vi "Waaagh_ProcessImage_Binary.vi"() -> ()   [LabVIEW 2016]
uses:
  <vilib>/vision/NI_Vision_Development_Module.lvlib
panel:
  out "Image 2":T1(plugin-control)
  out "Image":T1(plugin-control)
  in  "stop":bool
  in  "Binary":string
  in  "Range":cluster{"Lower value":sgl, "Upper value":sgl}={"Lower value"=128.0, "Upper value"=255.0} {"Upper value" format="%.2f"; "Lower value" format="%.2f"}
  in  "File Path":path
  in  "String":string
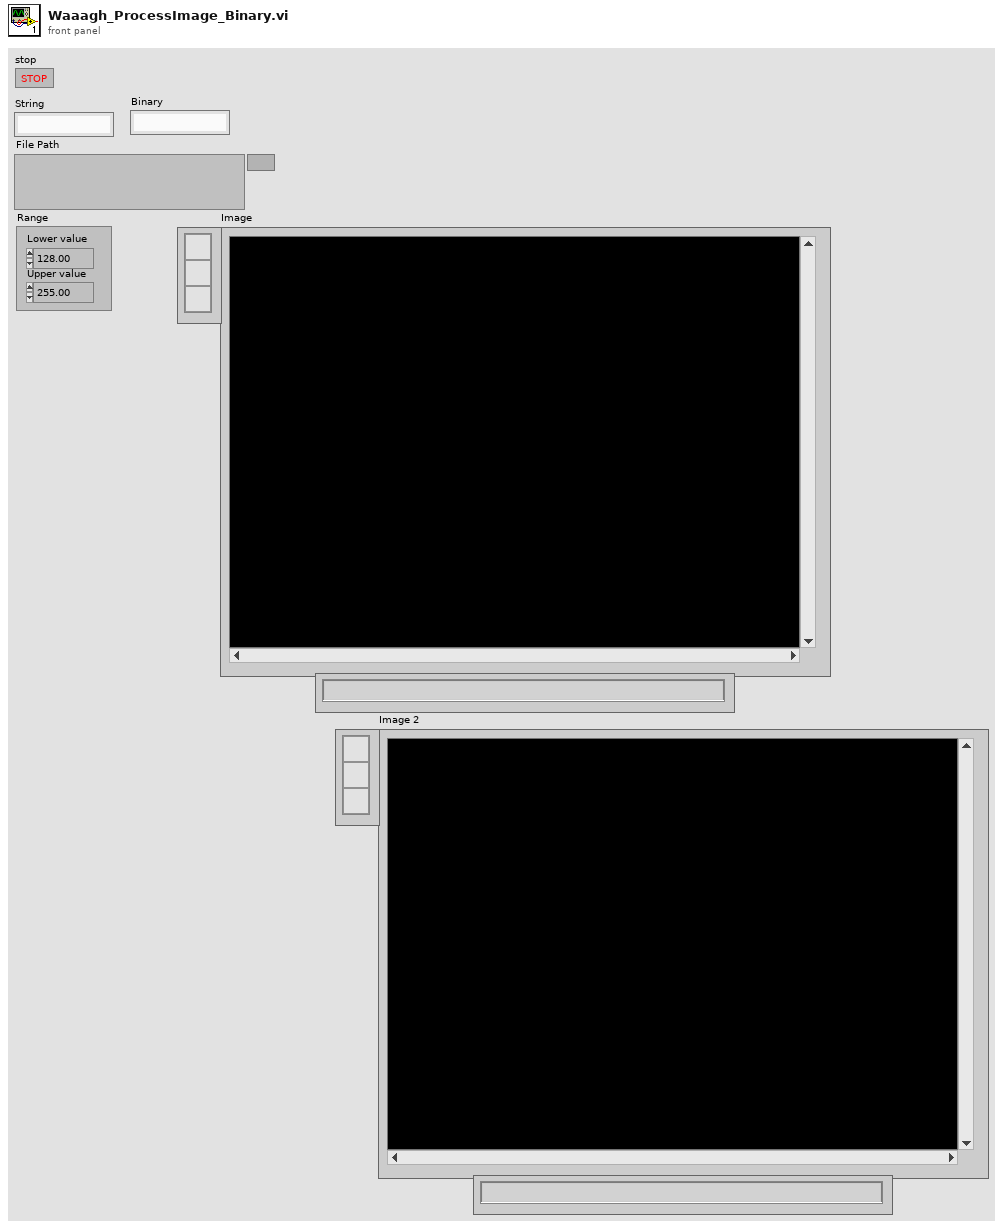
[diagram p1: front panel]
types:
  T1 = typedef "IMAQ Image.ctl" = refnum<image>
  T2 = typedef "Image Type" = u32
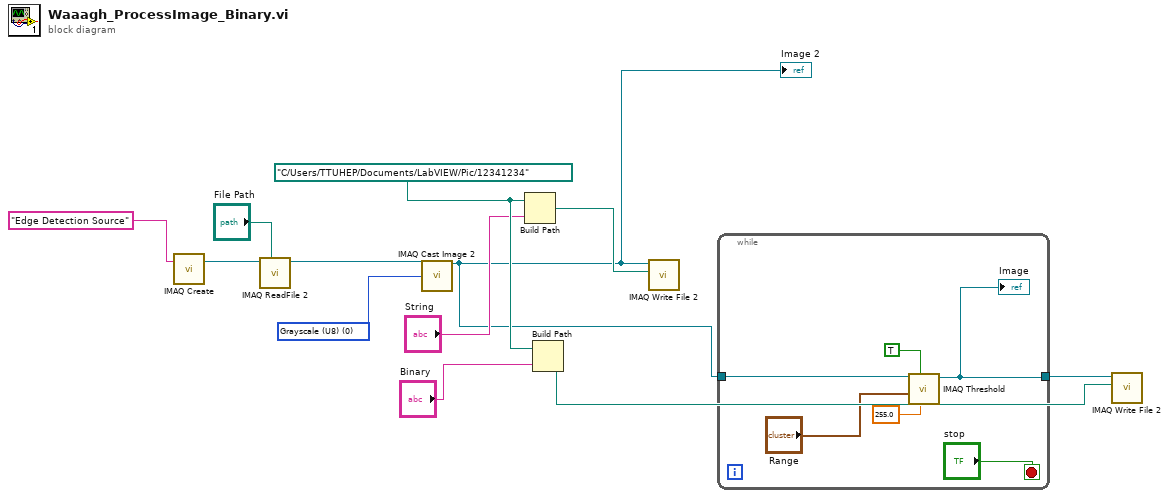
[diagram p0: block diagram]
diagram:
  w6 = path "C:/Users/TTUHEP/Documents/LabVIEW/Pic/12341234"
  w12 = T2 0 items=["Grayscale (U8)", "Grayscale (I16)", "Grayscale (SGL)", "Complex (CSG)", "RGB (U32)", "HSL (U32)", "RGB (U64)", "Grayscale (U16)"] ("Image Type")
  n1 = call "IMAQ Create"("Image Name"="Edge Detection Source") -> ("New Image"=w9:T1)  [unwired: 4 in, 1 out]
  n2 = call "IMAQ ReadFile 2"("File Path"="File Path", "Image"=w9) -> ("Image Out"=w8:T1)  [unwired: 5 in, 4 out]
  n3 = call "IMAQ Cast Image 2"("Image Src"=w8, "Image Type"=w12) -> ("Image Dst Out"=w1:T1)  [unwired: 12 in, 1 out]
  "Image 2" <- w1
  n4 = Build Path(base path=w6, name or relative path="String") -> (appended path=w11:path)
  n5 = Build Path(base path=w6, name or relative path="Binary") -> (appended path=w3:path)
  n6 = call-poly "IMAQ Write File 2"("File Path"=w11, "Image"=w1) -> ()  [unwired: 8 in, 2 out]
  n7 = while {
    tunnel: w1 -> [w18]
    tunnel: [w15] -> w4
    stop <- "stop" stop-if-true
    n8 = call "IMAQ Threshold"("Replace Value"=sgl 255.0, "Keep/Replace Value (Replace)"=TRUE, "Range"="Range", "Image Src"=w18) -> ("Image Dst Out"=w15:T1)  [unwired: 6 in, 1 out]
    "Image" <- w15
  }
  n9 = call-poly "IMAQ Write File 2"("File Path"=w3, "Image"=w4) -> ()  [unwired: 8 in, 2 out]
